vi "libdaq_adc_singleSample.vi"(0 "error in (no error)":errorcluster, 1 "device_name":string, 2 "module_name":string, 4 "channelist":u8[](array[numeric])) -> (14 "error out":errorcluster, 15 "device_name":string, 16 "module_name":string, 18 "resultbuf":dbl[](array[numeric]))   [LabVIEW 2010, in "libdaqVI.lvlib"]
doc: "ADC单次采样，根据采样通道数组channellist中的通道顺序，对每个通道进行单次采样，采样通道数组中的所有通道采集完成后返回采集结果"
uses:
  libdaqVI.lvlib
  dll/daqlib.dll
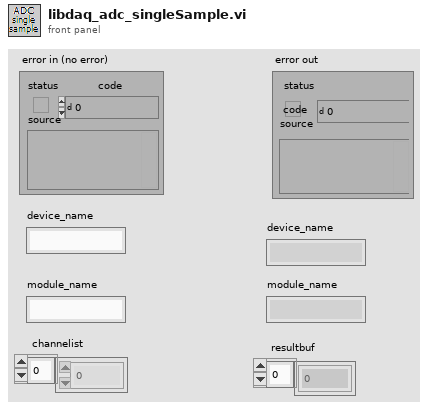
[diagram p1: front panel]
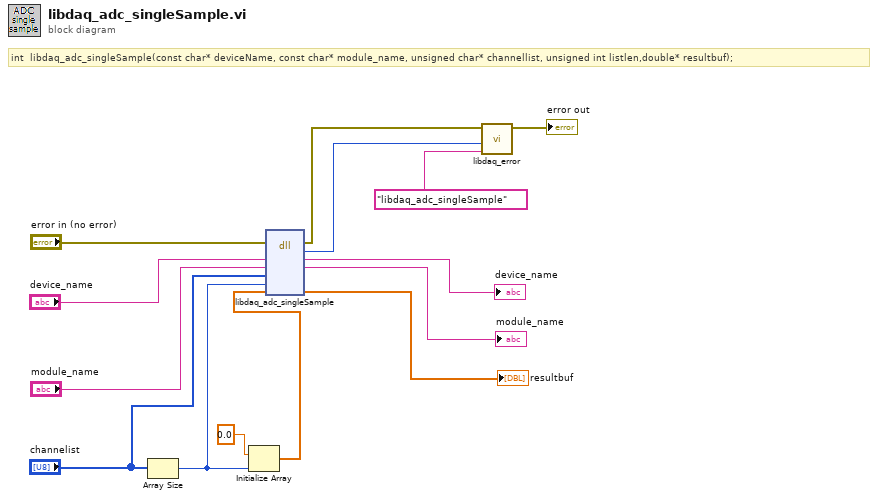
[diagram p0: block diagram]
diagram:
  # "int  libdaq_adc_singleSample(const char* deviceName, const char* module_name, unsigned char* channellist, unsigned int listlen,double* resultbuf);"
  n1 = Array Size(array="channelist") -> (size(s)=w7:i32)
  n2 = Initialize Array(0.0, w7) -> (w9:dbl[])
  n3 = dll-call lib="E:/Product/Example/DAQ-USB3212/Labview/labview_2010/libdaqVI/dll/daqlib.dll" fn="libdaq_adc_singleSample"(error in="error in (no error)", "device_name"="device_name", "module_name"="module_name", "channellist"="channelist", "listlen"=w7, "resultbuf"=w9) -> (error out=w4:errorcluster, "return type"=w2:i32, "device_name"=→"device_name":string, "module_name"=→"module_name":string, "resultbuf"=→"resultbuf":dbl[])  [unwired: 4 in, 1 out]
  n4 = call "libdaq_error.vi"("error source"="libdaq_adc_singleSample", "error code"=w2, "错误输入（无错误）"=w4) -> ("错误输出"=→"error out":errorcluster)  [unwired: 8 in]
